vi "2-city_section.vi"() -> ()   [LabVIEW 2015]
uses:
  class/Car.lvclass
panel:
  in  "Instructions":i32[][](array[numeric])
  out "Car.lvclass 2":refnum<class "Car.lvclass">
  in  "Car.lvclass":refnum<class "Car.lvclass">
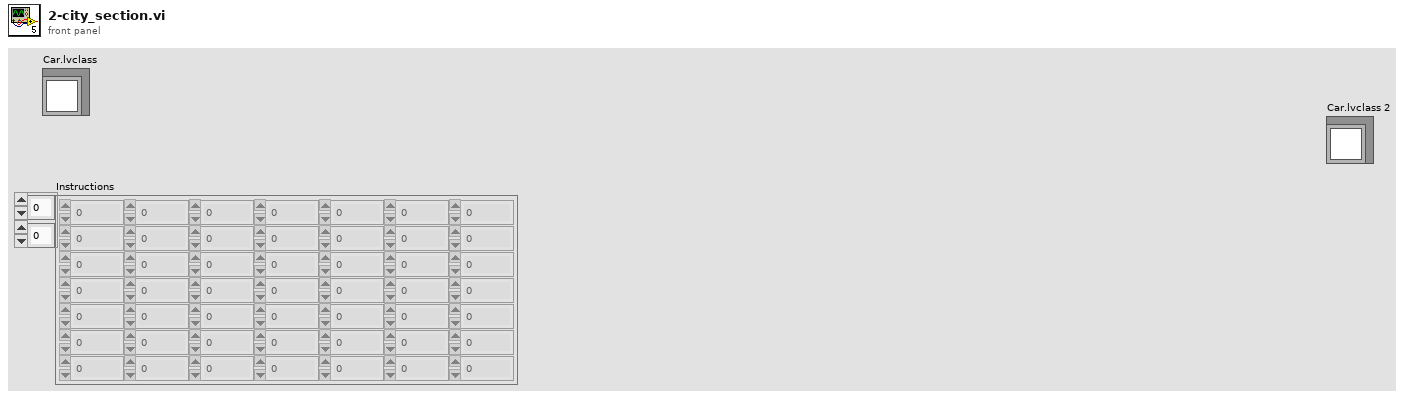
[diagram p1: front panel]
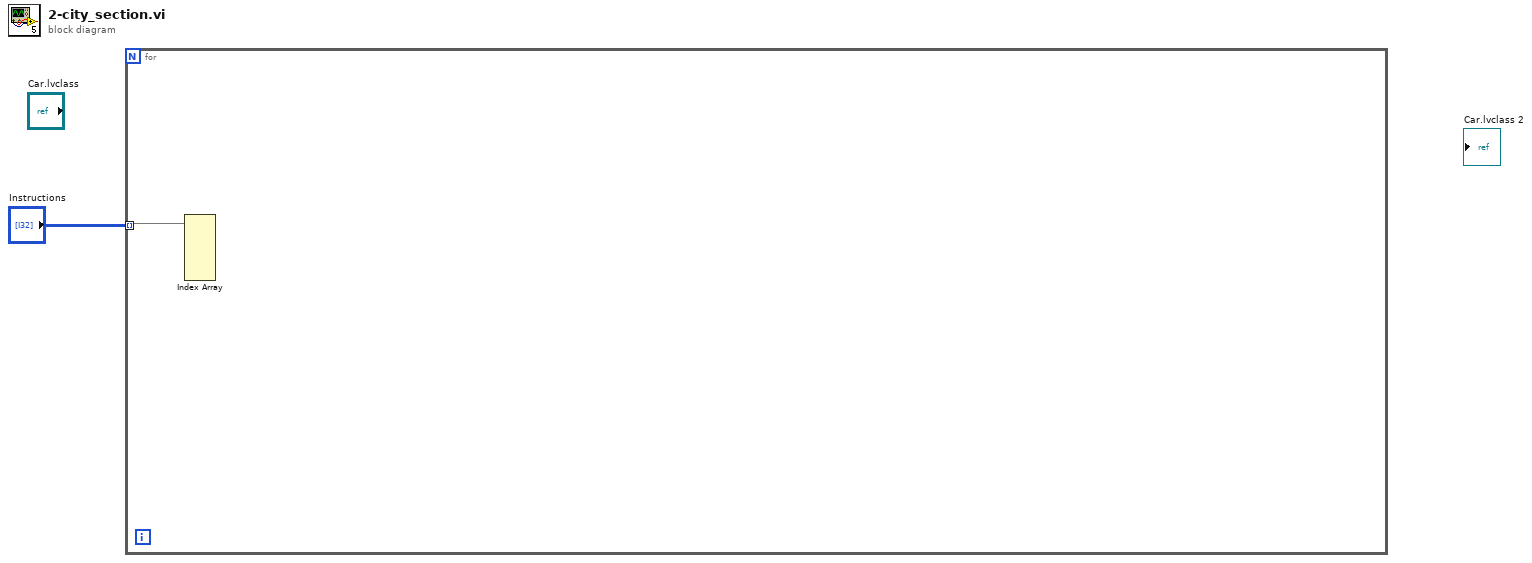
[diagram p0: block diagram]
diagram:
  n1 = for {
    tunnel: "Instructions" -> [w2] mode=indexing
    n2 = Index Array(array=w2) -> ()  [unwired: 6 in, 6 out]
  }
